vi "getViBookmarksInfo.vi"(8 "error in (no error)":errorcluster, 11 "VI in":refnum<vi>) -> (0 "error out":errorcluster, 2 "Bookmarks":string[][](array[string]), 3 "VI out":refnum<vi>)   [LabVIEW 2017, in "vi_tools.lvlib"]
doc: "Returns the bookmark information for the specified VI reference."
uses:
  066db6f1-c9bf-4861-a7de-4d1c13d50b6c.vi
  <vilib>/Utility/error.llb/Clear Errors.vi
  vi_tools.lvlib
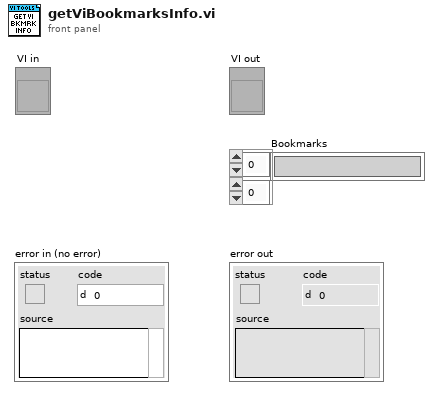
[diagram p1: front panel]
types:
  T1 = typedef "LVBookmarkInfoTypeDef.ctl" = cluster{"Bookmark Reference":u32, "Bookmark Tag":string, "Label Text":string}[]
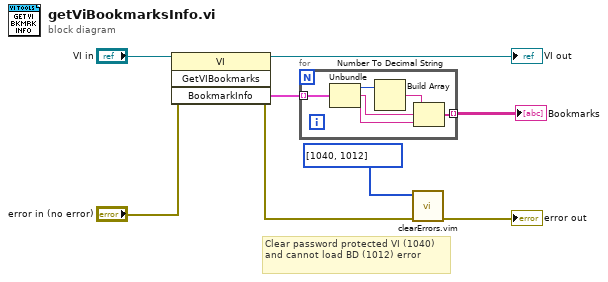
[diagram p0: block diagram]
diagram:
  # "Clear password protected VI (1040) and cannot load BD (1012) error"
  n1 = invoke class="VI" method="GetVIBookmarks"(reference="VI in", error in="error in (no error)") -> (reference out=→"VI out":refnum<vi>, error out=w3:errorcluster, "BookmarkInfo"=w5:T1)  [unwired: 2 in, 1 out]
  n2 = for {
    tunnel: w5 -> [w14] mode=indexing
    tunnel: [w9] -> w4 mode=indexing
    n3 = Unbundle(w14) -> ("Bookmark Reference"=w13:u32, "Bookmark Tag"=w11:string, "Label Text"=w10:string)
    n4 = Number To Decimal String(number=w13) -> (decimal integer string=w12:string)  [unwired: 1 in]
    n5 = Build Array(w12, w11, w10) -> (w9:string[])
  }
  "Bookmarks" <- w4
  n6 = call "clearErrors.vim"("Error in"=w3, "Specific Error Code to Clear"=i32[] [1040, 1012]) -> ("Error out"=→"error out":errorcluster)  [unwired: 8 in, 1 out]
